vi "CoboltLaser_AreYouThere.vi"(0 "ComPort":refnum<visa-resource-name>, 3 "GenerateError":bool=TRUE, 7 "error in (no error)":errorcluster) -> (20 "ComPortOut":refnum<visa-resource-name>, 23 "Connected":bool, 27 "error out":errorcluster)   [LabVIEW 2019]
doc: "Use this template to build a VI to use as a subVI."
panel:
  out "ResponseOK":bool
  out "Response":string
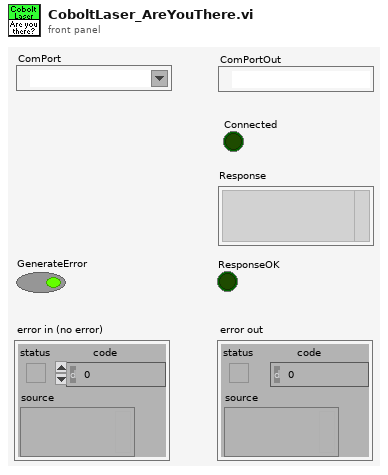
[diagram p1: front panel]
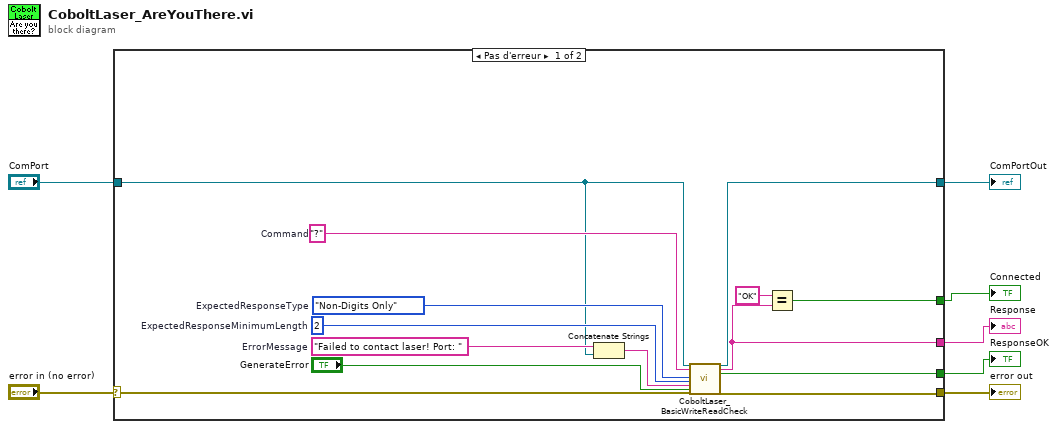
[diagram p0: block diagram]
diagram:
  n1 = case shown="Pas d'erreur" "error in (no error)" {
    selector: "error in (no error)" -> [w21 w23]
    tunnel: [w20 w23] -> w6
    tunnel: "ComPort" -> [w13 w22]
    tunnel: [w12 w22] -> w4
    tunnel: [w10 _] -> w3
    tunnel: [w9 _] -> w2
    tunnel: [w8 _] -> w1
    frame No Error {
      w17 = 2  # ExpectedResponseMinimumLength
      w18 = enum16{"Any", "Digits Only", "Non-Digits Only"}."Non-Digits Only"  # ExpectedResponseType
      w15 = "Failed to contact laser! Port: "  # ErrorMessage
      w19 = "?"  # Command
      n2 = Concatenate Strings(w15, w13) -> (w14:string)
      n3 = call <userlib>:"CoboltLaser_BasicWriteReadCheck.vi"("ComPort"=w13, "Command"=w19, "ExpectedResponseType"=w18, "ExpectedResponseMinimumLength"=w17, "ErrorMessage"=w14, "GenerateError"="GenerateError", "error in (no error)"=w21) -> ("ComPortOut"=w12:refnum<visa-resource-name>, "Response"=w8:string, "ResponseOK"=w9:bool, "error out"=w20:errorcluster)  [unwired: 17 in]
      n4 = Equal?(x="OK", y=w8) -> (x = y?=w10:bool)
    }
    frame Error {
    }
  }
  "error out" <- w6
  "ComPortOut" <- w4
  "Connected" <- w3
  "Response" <- w1
  "ResponseOK" <- w2
